vi "Write Content.vi"(8 "Error In":errorcluster, 10 "Content":string, 11 "Contentable In":refnum<class "Contentable.lvclass">) -> (0 "Error Out":errorcluster, 3 "Contentable Out":refnum<class "Contentable.lvclass">)   [LabVIEW 2018]
uses:
  Contentable.lvclass
  D:/Users/cfield/Code/Field R&D Services/Mustache/trunk/src/Toolkit/Low-Level/Tokens/Abstract/Abstract.lvclass
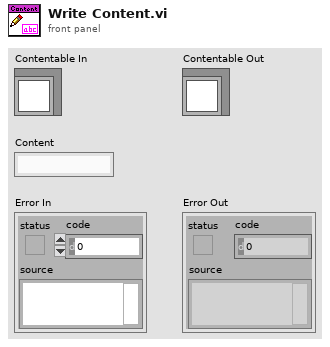
[diagram p1: front panel]
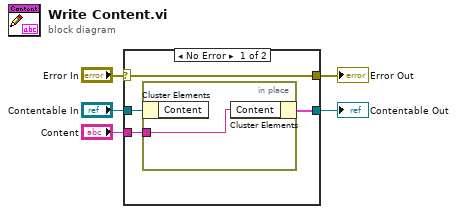
[diagram p0: block diagram]
diagram:
  n1 = case shown="No Error" "Error In" {
    selector: "Error In" -> [w9 w12]
    tunnel: [w9 w12] -> w4
    tunnel: [w6 w11] -> w2
    tunnel: "Contentable In" -> [w8 w11]
    tunnel: "Content" -> [w7 _]
    frame No Error {
      n2 = in-place {
        in-place-border: w7 -> [w10]
        n3 = in-place-cluster #1(w8) -> ()  [unwired: 1 out]
        n4 = in-place-cluster #1("Content"=w10) -> (w6:cluster{})
      }
    }
    frame Error {
    }
  }
  "Error Out" <- w4
  "Contentable Out" <- w2
